vi "EMI_project_v5.vi"() -> ()   [LabVIEW 2020]
uses:
  <vilib>/Instr/_visa.llb/VISA Flush IO Buffer Mask.ctl
  <vilib>/Analysis/baseanly.llb/Mean (DBL).vi
  <vilib>/Instr/_visa.llb/VISA Configure Serial Port (Instr).vi
  <vilib>/Analysis/NI_AALBase.lvlib
panel:
  out "Numeric 2":dbl
  out "Numeric":dbl
  out "Boolean":bool
  out "Auto Mix LED":bool
  in  "stop 4":bool
  in  "stop 3":bool
  out "V_avg_live_CH02":dbl
  out "V_avg_live_CH01":dbl
  in  "Auto Mix ON/OFF":bool
  out "Take Average CH02":bool
  out "Take Average CH01":bool
  in  "Take Average CH 01":bool
  out "Voltage Peak CH02":dynamicdata(graph)
  out "Voltage Peak CH01":dynamicdata(graph)
  in  "stop 2":bool
  out "Voltage Thresould\n CH 2":dbl
  in  "Noise Thresould \nCH02":dbl
  in  "Take Average CH 2":bool
  out "Voltage Thresould\n CH 01":dbl
  in  "Noise Thresould\n CH01":dbl
  out "Fader 02 level":dbl
  out "Fader 01 level":dbl
  out "Gain Knob 02 level":dbl
  out "Gain knob 01 level":dbl
  out "manual mode led":bool
  out "Sound Balance Mode":bool
  in  "Gain Knob 02":dbl(knob) scale=0.0..300.0
  in  "Gain Knob 01":dbl(knob) scale=0.0..300.0
  in  "Fader 02 Slider":dbl(slide) scale=0.0..10.0
  in  "Fader 01 Slider":dbl(slide) scale=0.0..10.0
  out "Fader 02 Max":dbl
  out "Fader 01 Max":dbl
  in  "Calibrate":bool
  in  "stop":bool
  in  "VISA Resource":refnum<visa-resource-name>
  in  "?":bool
  in  "Gain 02":bool
  in  "?":bool
  in  "Gain 01":bool
  in  "?":bool
  in  "Fader 02":bool
  in  "?":bool
  in  "Fader 01":bool
  # "Automation System For Analog Audio Mixers"
  # "Calibration \nMode"
  # "Manual Mode"
  # "Sound Balance Mode"
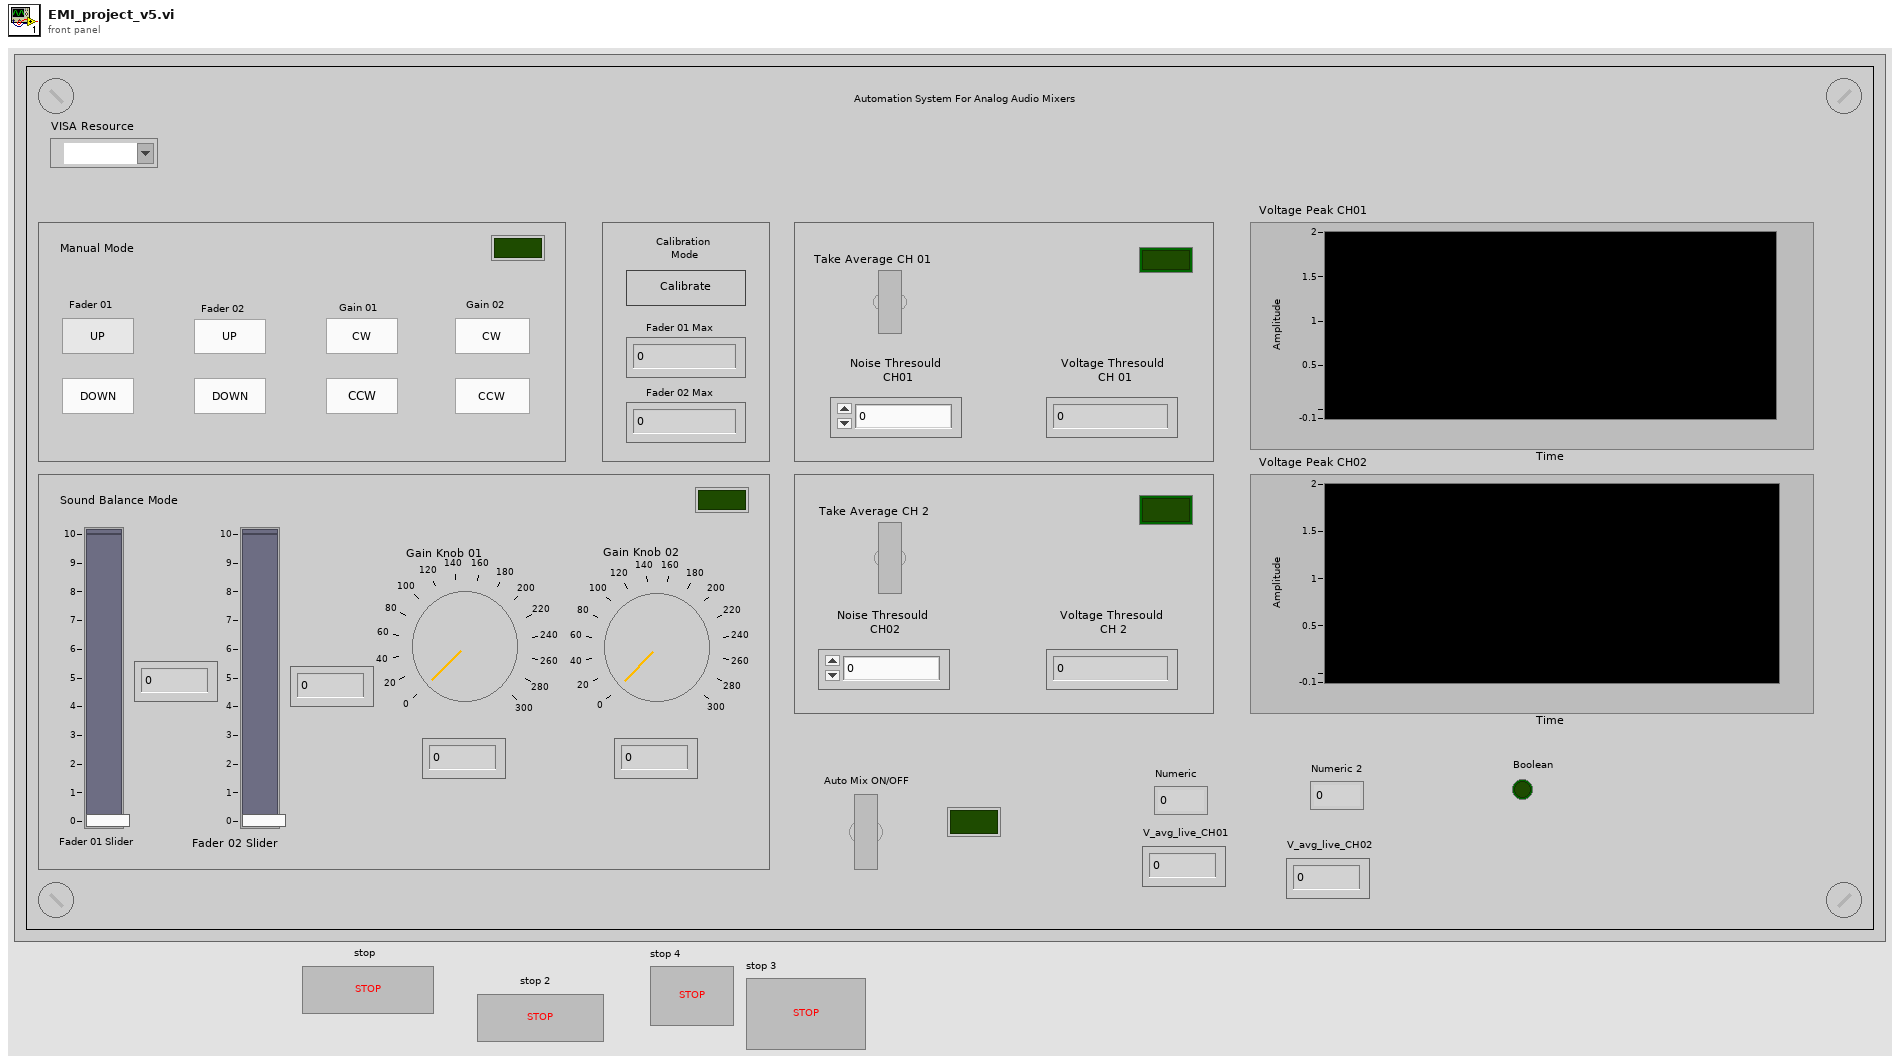
[diagram p1: front panel]
types:
  T1 = cluster{"Fader_Target_mm_1":dbl, "Fader_Target_mm_2":dbl, "Gain_Target_deg_1":dbl, "Gain_Target_deg_2":dbl}
  T2 = typedef "VISA Flush IO Buffer Mask.ctl" = u16
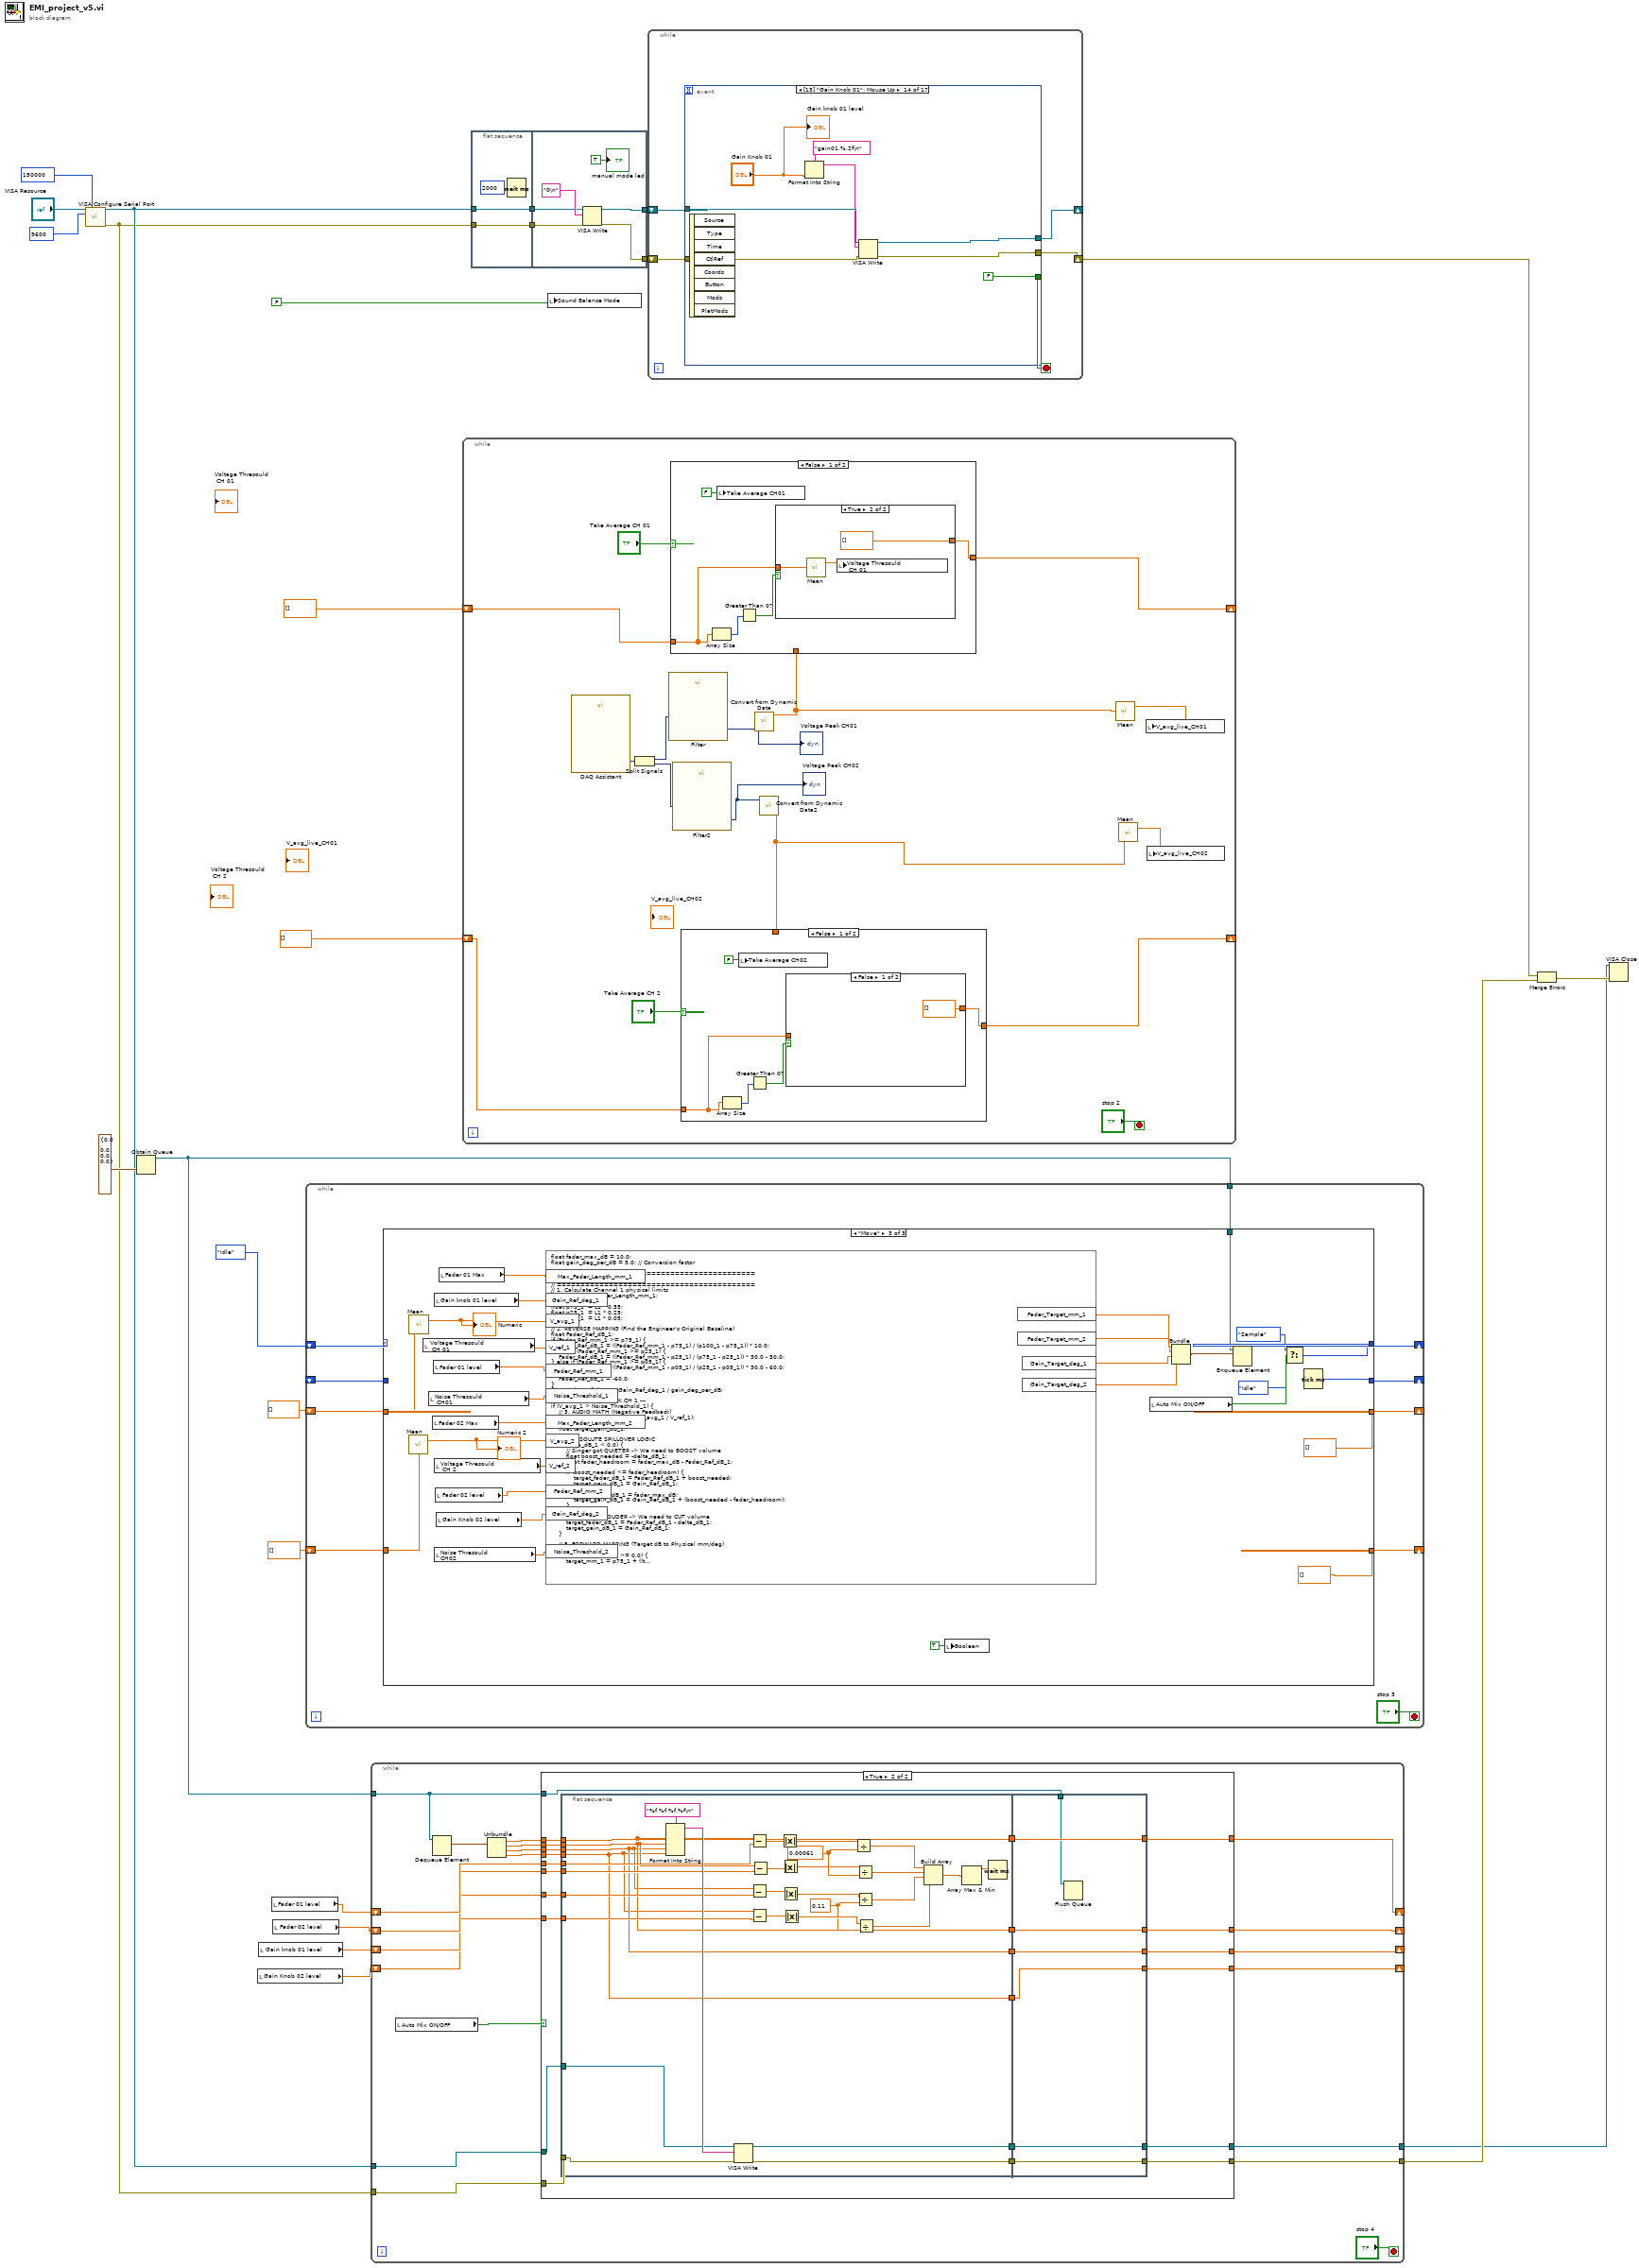
[diagram p0: block diagram]
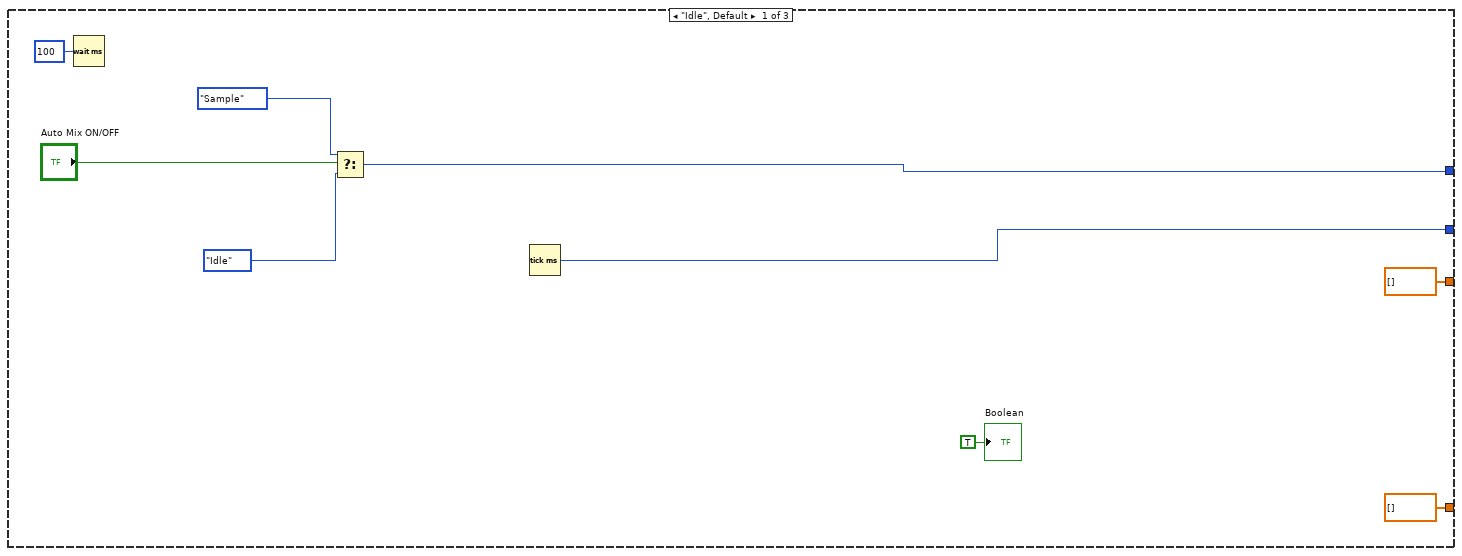
[diagram p3: hidden frame]
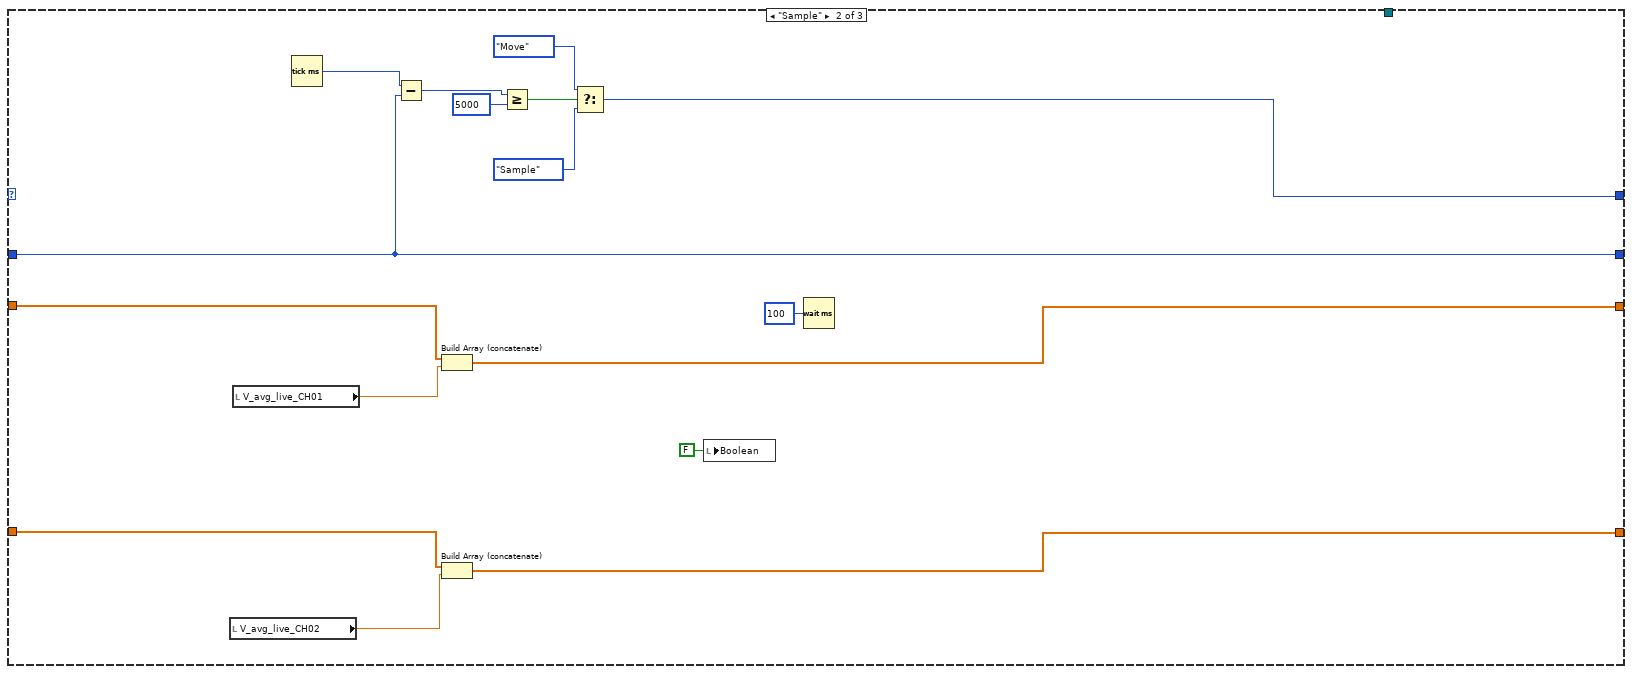
[diagram p4: hidden frame]
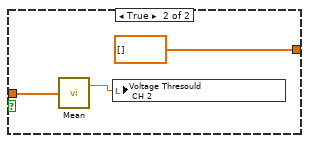
[diagram p5: hidden frame]
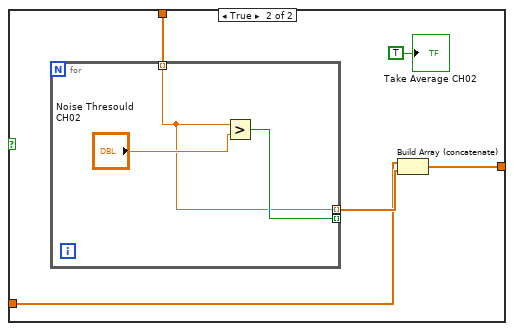
[diagram p6: hidden frame]
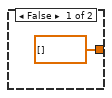
[diagram p7: hidden frame]
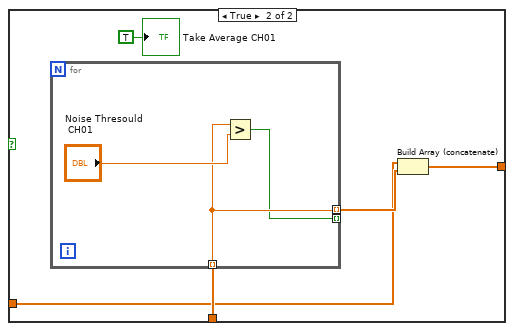
[diagram p8: hidden frame]
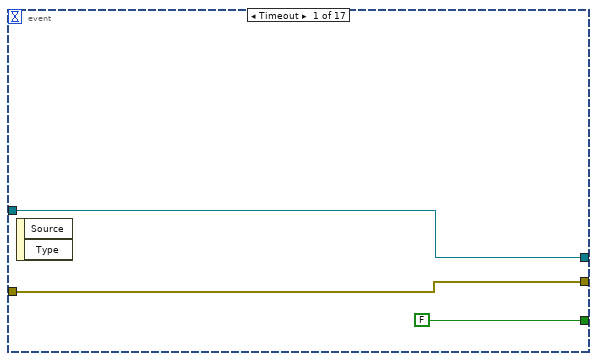
[diagram p9: hidden frame]
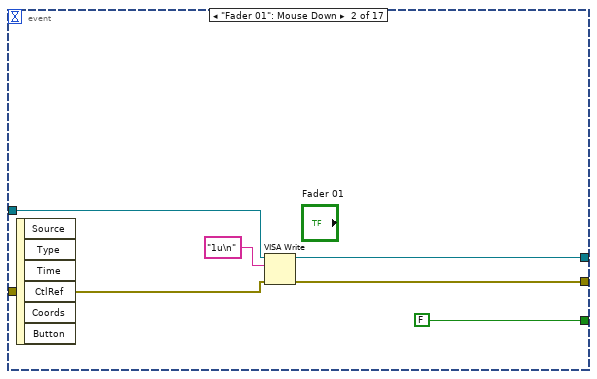
[diagram p10: hidden frame]
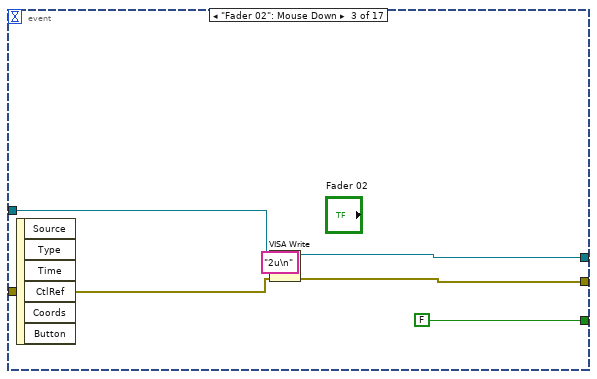
[diagram p11: hidden frame]
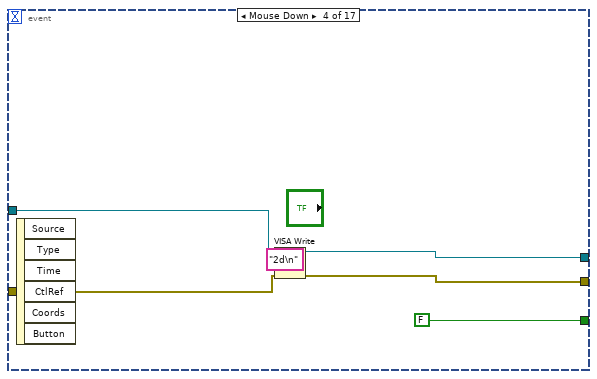
[diagram p12: hidden frame]
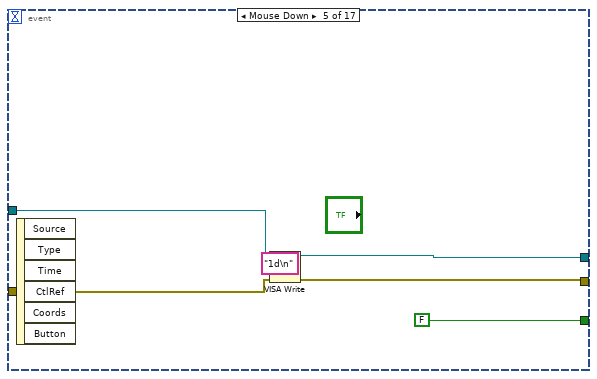
[diagram p13: hidden frame]
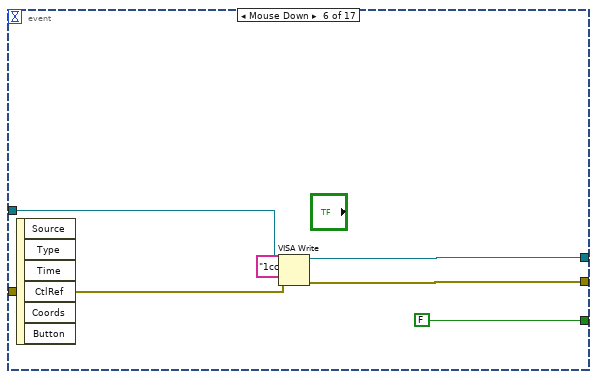
[diagram p14: hidden frame]
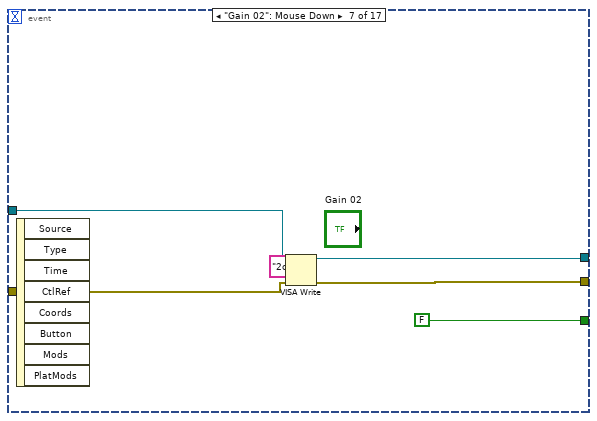
[diagram p15: hidden frame]
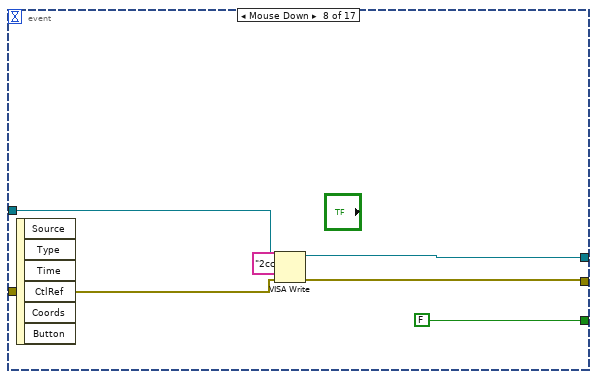
[diagram p16: hidden frame]
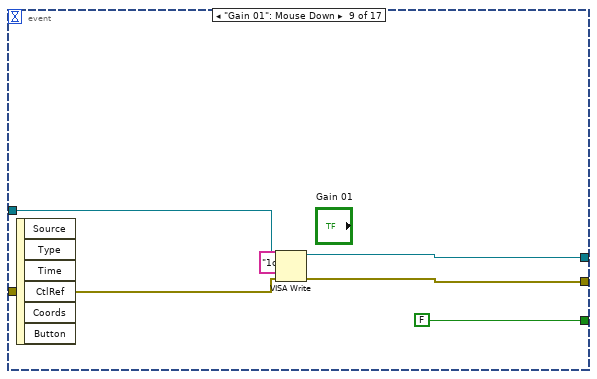
[diagram p17: hidden frame]
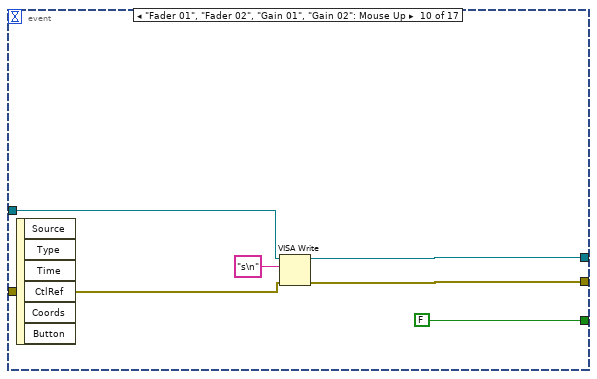
[diagram p18: hidden frame]
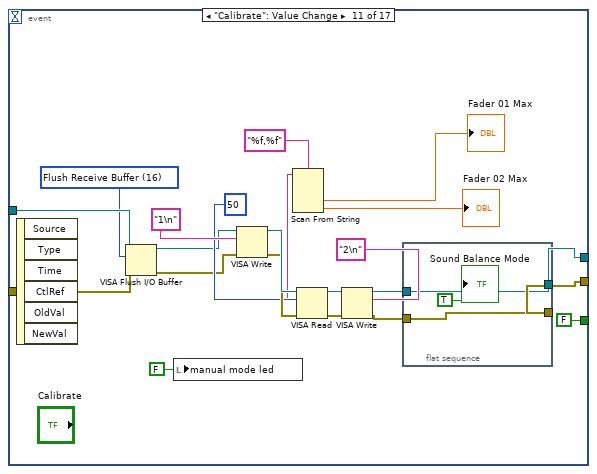
[diagram p19: hidden frame]
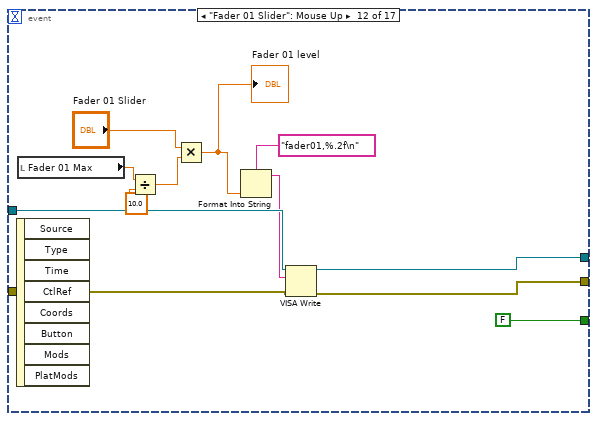
[diagram p20: hidden frame]
diagram:
  n1 = call-poly "VISA Configure Serial Port"("VISA resource name"="VISA Resource", "timeout (10sec)"=u32 150000, "baud rate (9600)"=u32 9600) -> ("VISA resource name out"=w11:refnum<visa-resource-name>, "error out"=w10:errorcluster)  [unwired: 11 in]
  n2 = Obtain Queue(element data type=T1 {"Fader_Target_mm_1"=0.0, "Fader_Target_mm_2"=0.0, "Gain_Target_deg_1"=0.0, "Gain_Target_deg_2"=0.0} ("output cluster")) -> (queue out=w12:refnum<queue>)  [unwired: 4 in, 2 out]
  n3 = local read "Gain Knob 02 level"() -> (w6:dbl)
  n4 = local read "Gain knob 01 level"() -> (w7:dbl)
  n5 = local read "Fader 01 level"() -> (w9:dbl)
  n6 = local read "Fader 02 level"() -> (w8:dbl)
  n7 = while {
    shift-right: [w34] -> _
    shift-left: enum16{"Idle", "Sample", "Move"}."Idle" -> [w35]
    shift-right: [w33] -> _
    shift-left: _ -> [w32]
    shift-right: [w30] -> _
    shift-left: dbl[] [] -> [w31]
    shift-right: [w29] -> _
    shift-left: dbl[] [] -> [w28]
    tunnel: w12 -> [w26]
    stop <- "stop 3" stop-if-true
    n8 = case shown="\"Move\"" w35 {
      tunnel: [w41 w54 w68] -> w34
      tunnel: [w36 w58 w63] -> w33
      tunnel: w32 -> [_ w58 _]
      tunnel: w31 -> [_ w53 w88]
      tunnel: [dbl[] [] w51 dbl[] []] -> w30
      tunnel: [dbl[] [] w48 dbl[] []] -> w29
      tunnel: w28 -> [_ w47 w85]
      tunnel: w26 -> [_ _ w73]
      frame "Idle", Default {
        n9 = Wait (ms)(milliseconds to wait=u32 100) -> ()  [unwired: 1 out]
        n10 = Select(t=enum16{"Idle", "Sample", "Move", "Wait"}."Sample", s="Auto Mix ON/OFF", f=enum16{"Idle", "Sample", "Move", "Wait"}."Idle") -> (s? t:f=w41:enum16{"Idle", "Sample", "Move", "Wait"})
        n11 = Tick Count (ms)() -> (millisecond timer value=w36:u32)
        "Boolean" <- TRUE ("Boolean")
      }
      frame "Sample" {
        n12 = local read "V_avg_live_CH02"() -> (w49:dbl)
        n13 = local read "V_avg_live_CH01"() -> (w52:dbl)
        n14 = Tick Count (ms)() -> (millisecond timer value=w45:u32)
        n15 = Subtract(x=w45, y=w58) -> (x-y=w60:u32)
        n16 = Build Array (concatenate)(w53, w52) -> (w51:dbl[])
        n17 = Build Array (concatenate)(w47, w49) -> (w48:dbl[])
        n18 = Greater Or Equal?(x=w60, y=u32 5000) -> (x >= y?=w57:bool)
        n19 = Select(t=enum16{"Idle", "Sample", "Move", "Wait"}."Move", s=w57, f=enum16{"Idle", "Sample", "Move", "Wait"}."Sample") -> (s? t:f=w54:enum16{"Idle", "Sample", "Move", "Wait"})
        n20 = local write "Boolean"(FALSE ("Boolean")) -> ()
        n21 = Wait (ms)(milliseconds to wait=u32 100) -> ()  [unwired: 1 out]
      }
      frame "Move" {
        n22 = call-poly <vilib>:"Mean.vi"("X"=w85) -> ("mean"=w61:dbl)  [unwired: 1 out]
        "Numeric 2" <- w61
        n23 = call-poly <vilib>:"Mean.vi"("X"=w88) -> ("mean"=w62:dbl)  [unwired: 1 out]
        "Numeric" <- w62
        n24 = local read "Voltage Thresould\n CH 01"() -> (w83:dbl)
        n25 = local read "Noise Thresould\n CH01"() -> (w66:dbl)
        n26 = local read "Fader 02 Max"() -> (w67:dbl)
        n27 = local read "Fader 01 level"() -> (w81:dbl)
        n28 = local read "Gain knob 01 level"() -> (w80:dbl)
        n29 = local read "Voltage Thresould\n CH 2"() -> (w82:dbl)
        n30 = local read "Noise Thresould \nCH02"() -> (w65:dbl)
        n31 = local read "Fader 02 level"() -> (w79:dbl)
        n32 = local read "Gain Knob 02 level"() -> (w78:dbl)
        n33 = local read "Fader 01 Max"() -> (w84:dbl)
        n34 = formula code="float fader_max_dB = 10.0;\nfloat gain_deg_per_dB = 5.0; // Conversion factor\n\n// ==========================================\n// CHANNEL 1 PROCESSING\n// ==========================================\n// 1. Calculate Channel 1 physical limits\nfloat L1 = Max_Fader_Length_mm_1; \nfloat p100_1 = L1;           \nfloat p75_1  = L1 * 0.55;    \nfloat p25_1  = L1 * 0.25;    \nfloat p05_1  = L1 * 0.05;    \n\n// 2. REVERSE MAPPING (Find the Engineer's Original Baseline)\nfloat Fader_Ref_dB_1;\nif (Fader_Ref_mm_1 >= p75_1) {\n    Fader_Ref_dB_1 = ((Fader_Ref_mm_1 - p75_1) / (p100_1 - p75_1)) * 10.0;\n} else if (Fader_Ref_mm_1 >= p25_1) {\n    Fader_Ref_dB_1 = ((Fader_Ref_mm_1 - p25_1) / (p75_1 - p25_1)) * 30.0 - 30.0;\n} else if (Fader_Ref_mm_1 >= p05_1) {\n    Fader_Ref_dB_1 = ((Fader_Ref_mm_1 - p05_1) / (p25_1 - p05_1)) * 30.0 - 60.0;\n} else {\n    Fader_Ref_dB_1 = -60.0; \n}\nfloat Gain_Ref_dB_1 = Gain_Ref_deg_1 / gain_deg_per_dB;\n\n// --- NOISE GATE CHECK CH 1 ---\nif (V_avg_1 > Noise_Threshold_1) {\n    // 3. AUDIO MATH (Negative Feedback)\n    float delta_dB_1 = 20 * log(V_avg_1 / V_ref_1);\n    float target_fader_dB_1;\n    float target_gain_dB_1;\n\n    // 4. ABSOLUTE SPILLOVER LOGIC\n    if (delta_dB_1 < 0.0) {\n        // Singer got QUIETER -> We need to BOOST volume\n        float boost_needed = -delta_dB_1; \n        float fader_headroom = fader_max_dB - Fader_Ref_dB_1;\n        \n        if (boost_needed <= fader_headroom) {\n            target_fader_dB_1 = Fader_Ref_dB_1 + boost_needed;\n            target_gain_dB_1 = Gain_Ref_dB_1;\n        } else {\n            target_fader_dB_1 = fader_max_dB;\n            target_gain_dB_1 = Gain_Ref_dB_1 + (boost_needed - fader_headroom);\n        }\n    } else {\n        // Singer got LOUDER -> We need to CUT volume\n        target_fader_dB_1 = Fader_Ref_dB_1 - delta_dB_1;\n        target_gain_dB_1 = Gain_Ref_dB_1;\n    }\n\n    // 5. FORWARD MAPPING (Target dB to Physical mm/deg)\n    float target_mm_1;\n    if (target_fader_dB_1 >= 0.0) {\n        target_mm_1 = p75_1 + ((target_fader_dB_1 - 0.0) / 10.0) * (p100_1 - p75_1);\n    } else if (target_fader_dB_1 >= -30.0) {\n        target_mm_1 = p25_1 + ((target_fader_dB_1 - (-30.0)) / 30.0) * (p75_1 - p25_1);\n    } else if (target_fader_dB_1 >= -60.0) {\n        target_mm_1 = p05_1 + ((target_fader_dB_1 - (-60.0)) / 30.0) * (p25_1 - p05_1);\n    } else {\n        target_mm_1 = 0.0; \n    }\n\n    Fader_Target_mm_1 = target_mm_1;\n    Gain_Target_deg_1 = target_gain_dB_1 * gain_deg_per_dB; \n\n    // 6. HARDWARE SAFETY CLAMP\n    if (Gain_Target_deg_1 > 300) { Gain_Target_deg_1 = 300; }\n    if (Gain_Target_deg_1 < 0.0) { Gain_Target_deg_1 = 0.0; }\n\n} else {\n    // AUDIO IS BELOW NOISE THRESHOLD\n    // Do nothing: lock the targets to the current physical positions\n    Fader_Target_mm_1 = Fader_Ref_mm_1;\n    Gain_Target_deg_1 = Gain_Ref_deg_1;\n}\n\n\n// ==========================================\n// CHANNEL 2 PROCESSING\n// ==========================================\n// 1. Calculate Channel 2 physical limits\nfloat L2 = Max_Fader_Length_mm_2; \nfloat p100_2 = L2;           \nfloat p75_2  = L2 * 0.55;    \nfloat p25_2  = L2 * 0.25;    \nfloat p05_2  = L2 * 0.05;    \n\n// 2. REVERSE MAPPING (Find the Engineer's Original Baseline)\nfloat Fader_Ref_dB_2;\nif (Fader_Ref_mm_2 >= p75_2) {\n    Fader_Ref_dB_2 = ((Fader_Ref_mm_2 - p75_2) / (p100_2 - p75_2)) * 10.0;\n} else if (Fader_Ref_mm_2 >= p25_2) {\n    Fader_Ref_dB_2 = ((Fader_Ref_mm_2 - p25_2) / (p75_2 - p25_2)) * 30.0 - 30.0;\n} else if (Fader_Ref_mm_2 >= p05_2) {\n    Fader_Ref_dB_2 = ((Fader_Ref_mm_2 - p05_2) / (p25_2 - p05_2)) * 30.0 - 60.0;\n} else {\n    Fader_Ref_dB_2 = -60.0; \n}\nfloat Gain_Ref_dB_2 = Gain_Ref_deg_2 / gain_deg_per_dB;\n\n// --- NOISE GATE CHECK CH 2 ---\nif (V_avg_2 > Noise_Threshold_2) {\n    // 3. AUDIO MATH (Negative Feedback)\n    float delta_dB_2 = 20 * log(V_avg_2 / V_ref_2);\n    float target_fader_dB_2;\n    float target_gain_dB_2;\n\n    // 4. ABSOLUTE SPILLOVER LOGIC\n    if (delta_dB_2 < 0.0) {\n        // Singer got QUIETER -> We need to BOOST volume\n        float boost_needed = -delta_dB_2; \n        float fader_headroom = fader_max_dB - Fader_Ref_dB_2;\n        \n        if (boost_needed <= fader_headroom) {\n            target_fader_dB_2 = Fader_Ref_dB_2 + boost_needed;\n            target_gain_dB_2 = Gain_Ref_dB_2;\n        } else {\n            target_fader_dB_2 = fader_max_dB;\n            target_gain_dB_2 = Gain_Ref_dB_2 + (boost_needed - fader_headroom);\n        }\n    } else {\n        // Singer got LOUDER -> We need to CUT volume\n        target_fader_dB_2 = Fader_Ref_dB_2 - delta_dB_2;\n        target_gain_dB_2 = Gain_Ref_dB_2;\n    }\n\n    // 5. FORWARD MAPPING (Target dB to Physical mm/deg)\n    float target_mm_2;\n    if (target_fader_dB_2 >= 0.0) {\n        target_mm_2 = p75_2 + ((target_fader_dB_2 - 0.0) / 10.0) * (p100_2 - p75_2);\n    } else if (target_fader_dB_2 >= -30.0) {\n        target_mm_2 = p25_2 + ((target_fader_dB_2 - (-30.0)) / 30.0) * (p75_2 - p25_2);\n    } else if (target_fader_dB_2 >= -60.0) {\n        target_mm_2 = p05_2 + ((target_fader_dB_2 - (-60.0)) / 30.0) * (p25_2 - p05_2);\n    } else {\n        target_mm_2 = 0.0; \n    }\n\n    Fader_Target_mm_2 = target_mm_2;\n    Gain_Target_deg_2 = target_gain_dB_2 * gain_deg_per_dB; \n\n    // 6. HARDWARE SAFETY CLAMP\n    if (Gain_Target_deg_2 > 300) { Gain_Target_deg_2 = 300; }\n    if (Gain_Target_deg_2 < 0.0) { Gain_Target_deg_2 = 0.0; }\n\n} else {\n    // AUDIO IS BELOW NOISE THRESHOLD\n    // Do nothing: lock the targets to the current physical positions\n    Fader_Target_mm_2 = Fader_Ref_mm_2;\n    Gain_Target_deg_2 = Gain_Ref_deg_2;\n}"("Max_Fader_Length_mm_1"=w84, "Max_Fader_Length_mm_2"=w67, "V_avg_1"=w62, "V_ref_1"=w83, "V_avg_2"=w61, "V_ref_2"=w82, "Fader_Ref_mm_1"=w81, "Fader_Ref_mm_2"=w79, "Gain_Ref_deg_1"=w80, "Gain_Ref_deg_2"=w78, "Noise_Threshold_1"=w66, "Noise_Threshold_2"=w65) -> ("Fader_Target_mm_1"=w77:dbl, "Fader_Target_mm_2"=w76:dbl, "Gain_Target_deg_1"=w75:dbl, "Gain_Target_deg_2"=w74:dbl)
        n35 = local write "Boolean"(TRUE ("Boolean")) -> ()
        n36 = local read "Auto Mix ON/OFF"() -> (w71:bool)
        n37 = Bundle("Fader_Target_mm_1"=w77, "Fader_Target_mm_2"=w76, "Gain_Target_deg_1"=w75, "Gain_Target_deg_2"=w74) -> (w72:T1)  [unwired: 1 in]
        n38 = Enqueue Element(queue=w73, element=w72) -> ()  [unwired: 2 in, 3 out]
        n39 = Select(t=enum16{"Idle", "Sample", "Move", "Wait"}."Sample", s=w71, f=enum16{"Idle", "Sample", "Move", "Wait"}."Idle") -> (s? t:f=w68:enum16{"Idle", "Sample", "Move", "Wait"})
        n40 = Tick Count (ms)() -> (millisecond timer value=w63:u32)
      }
    }
  }
  n41 = while {
    tunnel: w12 -> [w89]
    tunnel: w11 -> [w102]
    tunnel: w10 -> [w101]
    shift-right: [w96] -> _
    shift-left: w9 -> [w100]
    shift-right: [w95] -> _
    shift-left: w8 -> [w99]
    shift-right: [w94] -> _
    shift-left: w7 -> [w98]
    shift-right: [w93] -> _
    shift-left: w6 -> [w97]
    tunnel: [w92] -> w2
    tunnel: [w91] -> w5
    stop <- "stop 4" stop-if-true
    n42 = local read "Auto Mix ON/OFF"() -> (w107:bool)
    n43 = Dequeue Element(queue=w89) -> (element=w108:T1)  [unwired: 2 in, 3 out]
    n44 = Unbundle(w108) -> ("Fader_Target_mm_1"=w106:dbl, "Fader_Target_mm_2"=w105:dbl, "Gain_Target_deg_1"=w104:dbl, "Gain_Target_deg_2"=w103:dbl)
    n45 = case shown="True" w107 {
      tunnel: w106 -> [_ w137]
      tunnel: w105 -> [_ w136]
      tunnel: w104 -> [_ w135]
      tunnel: w103 -> [_ w134]
      tunnel: w102 -> [w110 w132]
      tunnel: w101 -> [w109 w133]
      tunnel: w100 -> [w114 w131]
      tunnel: w99 -> [w113 w130]
      tunnel: w98 -> [w112 w129]
      tunnel: w97 -> [w111 w128]
      tunnel: [w114 w126] -> w96
      tunnel: [w113 w125] -> w95
      tunnel: [w112 w123] -> w94
      tunnel: [w111 w120] -> w93
      tunnel: [w110 w119] -> w92
      tunnel: [w109 w117] -> w91
      tunnel: w89 -> [_ w115]
      frame False {
      }
      frame True {
        n46 = flat-sequence {
          tunnel: w137 -> [w145]
          tunnel: w136 -> [w144]
          tunnel: w135 -> [w143]
          tunnel: w134 -> [w142]
          tunnel: w133 -> [w138]
          tunnel: w132 -> [w139]
          tunnel: w131 -> [w165]
          tunnel: w130 -> [w164]
          tunnel: w129 -> [w163]
          tunnel: w128 -> [w162]
          tunnel: [w145] -> w127
          tunnel: [w144] -> w124
          tunnel: [w143] -> w122
          tunnel: [w142] -> w121
          tunnel: [w141] -> w118
          tunnel: [w140] -> w116
          tunnel: w127 -> [w174]
          tunnel: [w174] -> w126
          tunnel: [w173] -> w125
          tunnel: w124 -> [w173]
          tunnel: [w172] -> w123
          tunnel: w122 -> [w172]
          tunnel: w121 -> [w171]
          tunnel: [w171] -> w120
          tunnel: [w170] -> w119
          tunnel: w118 -> [w170]
          tunnel: [w169] -> w117
          tunnel: w116 -> [w169]
          tunnel: w115 -> [w168]
          frame #0 {
            w148 = 0.11 ("y")
            w157 = 0.00061 ("y")
            n47 = Format Into String(format string="%f,%f,%f,%f\n", w145, w144, w143, w142) -> (resulting string=w166:string)  [unwired: 2 in, 1 out]
            n48 = VISA Write(VISA resource name=w139, write buffer=w166, error in (no error)=w138) -> (VISA resource name out=w141:refnum<visa-resource-name>, error out=w140:errorcluster)  [unwired: 1 out]
            n49 = Subtract(x=w145, y=w165) -> (x-y=w161:dbl)
            n50 = Subtract(x=w143, y=w163) -> (x-y=w159:dbl)
            n51 = Subtract(x=w142, y=w162) -> (x-y=w158:dbl)
            n52 = Subtract(x=w144, y=w164) -> (x-y=w160:dbl)
            n53 = Absolute Value(x=w161) -> (abs(x)=w156:dbl)
            n54 = Absolute Value(x=w160) -> (abs(x)=w155:dbl)
            n55 = Absolute Value(x=w159) -> (abs(x)=w154:dbl)
            n56 = Absolute Value(x=w158) -> (abs(x)=w153:dbl)
            n57 = Divide(x=w156, y=w157) -> (x/y=w152:dbl)
            n58 = Divide(x=w155, y=w157) -> (x/y=w151:dbl)
            n59 = Divide(x=w154, y=w148) -> (x/y=w150:dbl)
            n60 = Divide(x=w153, y=w148) -> (x/y=w149:dbl)
            n61 = Build Array(w152, w151, w150, w149) -> (w147:dbl[])
            n62 = Array Max & Min(array=w147) -> (max value=w146:dbl)  [unwired: 3 out]
            n63 = Wait (ms)(milliseconds to wait=w146) -> ()  [unwired: 1 out]
          }
          frame #1 {
            n64 = Flush Queue(queue=w168) -> ()  [unwired: 1 in, 3 out]
          }
        }
      }
    }
  }
  n65 = while {
    shift-right: [w185] -> _
    shift-left: dbl[] [] -> [w186]
    shift-right: [w183] -> _
    shift-left: dbl[] [] -> [w182]
    stop <- "stop 2" stop-if-true
    n66 = call "DAQ Assistant"() -> ("data"=w189:dynamicdata)  [unwired: 16 in, 3 out]
    n67 = Split Signals(w189) -> (w188:dynamicdata, w187:dynamicdata)  [unwired: 2 in]
    n68 = call "Filter"("Signal"=w188) -> ("Filtered Signal"=w180:dynamicdata)  [unwired: 9 in, 1 out]
    "Voltage Peak CH01" <- w180
    n69 = call "Filter2"("Signal"=w187) -> ("Filtered Signal"=w179:dynamicdata)  [unwired: 9 in, 1 out]
    "Voltage Peak CH02" <- w179
    n70 = call "Convert from Dynamic Data"("Dynamic Data Type"=w180) -> ("Array"=w176:dbl[])  [unwired: 3 in]
    n71 = case shown="False" "Take Average CH 01" {
      tunnel: w176 -> [_ w221]
      tunnel: w186 -> [w210 w218]
      tunnel: [w209 w219] -> w185
      frame False {
        n72 = Array Size(array=w210) -> (size(s)=w212:i32)
        n73 = local write "Take Average CH01"(FALSE ("Take Average CH01")) -> ()
        n74 = Greater Than 0?(x=w212) -> (x > 0?=w211:bool)
        n75 = case shown="True" w211 {
          tunnel: w210 -> [_ w216]
          tunnel: [dbl[] [] dbl[] []] -> w209
          frame False {
          }
          frame True {
            n76 = call-poly <vilib>:"Mean.vi"("X"=w216) -> ("mean"=w215:dbl)  [unwired: 1 out]
            n77 = local write "Voltage Thresould\n CH 01"(w215) -> ()
          }
        }
      }
      frame True {
        n78 = for {
          tunnel: w221 -> [w223] mode=indexing
          tunnel: [w223] -> w220 mode=indexing if=w222
          tunnel: [w222] -> _ mode=indexing
          n79 = Greater?(x=w223, y="Noise Thresould\n CH01") -> (0:w222:bool)
        }
        n80 = Build Array (concatenate)(w218, w220) -> (w219:dbl[])
        "Take Average CH01" <- TRUE ("Take Average CH01")
      }
    }
    n81 = call "Convert from Dynamic Data2"("Dynamic Data Type"=w179) -> ("Array"=w175:dbl[])  [unwired: 3 in]
    n82 = case shown="False" "Take Average CH 2" {
      tunnel: w182 -> [w193 w203]
      tunnel: [w192 w202] -> w183
      tunnel: w175 -> [_ w201]
      frame False {
        n83 = Array Size(array=w193) -> (size(s)=w195:i32)
        n84 = local write "Take Average CH02"(FALSE ("Take Average CH02")) -> ()
        n85 = Greater Than 0?(x=w195) -> (x > 0?=w194:bool)
        n86 = case shown="False" w194 {
          tunnel: w193 -> [_ w199]
          tunnel: [dbl[] [] dbl[] []] -> w192
          frame False {
          }
          frame True {
            n87 = call-poly <vilib>:"Mean.vi"("X"=w199) -> ("mean"=w198:dbl)  [unwired: 1 out]
            n88 = local write "Voltage Thresould\n CH 2"(w198) -> ()
          }
        }
      }
      frame True {
        n89 = for {
          tunnel: [w205] -> w204 mode=indexing if=w206
          tunnel: [w206] -> _ mode=indexing
          tunnel: w201 -> [w205] mode=indexing
          n90 = Greater?(x=w205, y="Noise Thresould \nCH02") -> (0:w206:bool)
        }
        n91 = Build Array (concatenate)(w203, w204) -> (w202:dbl[])
        "Take Average CH02" <- TRUE ("Take Average CH02")
      }
    }
    n92 = call-poly <vilib>:"Mean.vi"("X"=w176) -> ("mean"=w178:dbl)  [unwired: 1 out]
    n93 = call-poly <vilib>:"Mean.vi"("X"=w175) -> ("mean"=w177:dbl)  [unwired: 1 out]
    n94 = local write "V_avg_live_CH01"(w178) -> ()
    n95 = local write "V_avg_live_CH02"(w177) -> ()
  }
  n96 = flat-sequence {
    tunnel: w10 -> [w226]
    tunnel: w11 -> [w227]
    tunnel: [w227] -> w21
    tunnel: [w226] -> w20
    tunnel: [w232] -> w23
    tunnel: [w231] -> w22
    tunnel: w21 -> [w230]
    tunnel: w20 -> [w229]
    frame #0 {
      n97 = Wait (ms)(milliseconds to wait=u32 2000) -> ()  [unwired: 1 out]
    }
    frame #1 {
      n98 = VISA Write(VISA resource name=w230, write buffer="0\n", error in (no error)=w229) -> (VISA resource name out=w232:refnum<visa-resource-name>, error out=w231:errorcluster)  [unwired: 1 out]
      "manual mode led" <- TRUE
    }
  }
  n99 = local write "Sound Balance Mode"(FALSE) -> ()
  n100 = while {
    shift-right: [w236] -> _
    shift-left: w23 -> [w238]
    shift-right: [w235] -> w4
    shift-left: w22 -> [w237]
    stop <- w234 stop-if-true
    n101 = event shown="[13] \"Gain Knob 01\": Mouse Up" {
      selector: _ -> [_ _ _ _ _ _ _ _ _ _ _ _ _ _ _ _ _]
      dyn-events: _ -> [_ _ _ _ _ _ _ _ _ _ _ _ _ _ _ _ _]
      timeout: _ -> [_ _ _ _ _ _ _ _ _ _ _ _ _ _ _ _ _]
      tunnel: w238 -> [w241 w247 w251 w257 w265 w268 w275 w281 w287 w293 w309 w327 w338 w351 w358 w364 w382]
      tunnel: w237 -> [w240 w246 w250 w256 w264 w269 w274 w280 w286 w292 w308 w326 w337 w350 w357 w362 w381]
      tunnel: [w241 w244 w253 w259 w262 w271 w277 w283 w289 w295 w300 w323 w335 w348 w355 w363 w382] -> w236
      tunnel: [w240 w243 w252 w258 w263 w270 w276 w282 w288 w294 w297 w325 w336 w349 w356 w361 w381] -> w235
      tunnel: [FALSE FALSE FALSE FALSE FALSE FALSE FALSE FALSE FALSE FALSE FALSE FALSE FALSE FALSE FALSE FALSE TRUE] -> w234
      event Timeout {
        n102 = event-data() -> ()  [unwired: 1 in, 2 out]
      }
      event "Fader 01": Mouse Down {
        n103 = event-data() -> ()  [unwired: 1 in, 6 out]
        n104 = VISA Write(VISA resource name=w247, write buffer="1u\n", error in (no error)=w246) -> (VISA resource name out=w244:refnum<visa-resource-name>, error out=w243:errorcluster)  [unwired: 1 out]
      }
      event "Fader 02": Mouse Down {
        n105 = event-data() -> ()  [unwired: 1 in, 6 out]
        n106 = VISA Write(VISA resource name=w251, write buffer="2u\n", error in (no error)=w250) -> (VISA resource name out=w253:refnum<visa-resource-name>, error out=w252:errorcluster)  [unwired: 1 out]
      }
      event Mouse Down {
        n107 = event-data() -> ()  [unwired: 1 in, 6 out]
        n108 = VISA Write(VISA resource name=w257, write buffer="2d\n", error in (no error)=w256) -> (VISA resource name out=w259:refnum<visa-resource-name>, error out=w258:errorcluster)  [unwired: 1 out]
      }
      event Mouse Down {
        n109 = event-data() -> ()  [unwired: 1 in, 6 out]
        n110 = VISA Write(VISA resource name=w265, write buffer="1d\n", error in (no error)=w264) -> (VISA resource name out=w262:refnum<visa-resource-name>, error out=w263:errorcluster)  [unwired: 1 out]
      }
      event Mouse Down {
        n111 = event-data() -> ()  [unwired: 1 in, 6 out]
        n112 = VISA Write(VISA resource name=w268, write buffer="1ccw\n", error in (no error)=w269) -> (VISA resource name out=w271:refnum<visa-resource-name>, error out=w270:errorcluster)  [unwired: 1 out]
      }
      event "Gain 02": Mouse Down {
        n113 = event-data() -> ()  [unwired: 1 in, 8 out]
        n114 = VISA Write(VISA resource name=w275, write buffer="2cw\n", error in (no error)=w274) -> (VISA resource name out=w277:refnum<visa-resource-name>, error out=w276:errorcluster)  [unwired: 1 out]
      }
      event Mouse Down {
        n115 = event-data() -> ()  [unwired: 1 in, 6 out]
        n116 = VISA Write(VISA resource name=w281, write buffer="2ccw\n", error in (no error)=w280) -> (VISA resource name out=w283:refnum<visa-resource-name>, error out=w282:errorcluster)  [unwired: 1 out]
      }
      event "Gain 01": Mouse Down {
        n117 = event-data() -> ()  [unwired: 1 in, 6 out]
        n118 = VISA Write(VISA resource name=w287, write buffer="1cw\n", error in (no error)=w286) -> (VISA resource name out=w289:refnum<visa-resource-name>, error out=w288:errorcluster)  [unwired: 1 out]
      }
      event "Fader 01", "Fader 02", "Gain 01", "Gain 02": Mouse Up {
        n119 = event-data() -> ()  [unwired: 1 in, 6 out]
        n120 = VISA Write(VISA resource name=w293, write buffer="s\n", error in (no error)=w292) -> (VISA resource name out=w295:refnum<visa-resource-name>, error out=w294:errorcluster)  [unwired: 1 out]
      }
      event "Calibrate": Value Change {
        w305 = T2 16 items=["Flush Receive Buffer"=16, "Write Transmit Buffer to Device"=32, "Flush Receive Buffer (No I/O)"=64, "Flush Transmit Buffer"=128] ("Mask")
        n121 = event-data() -> ()  [unwired: 1 in, 6 out]
        n122 = VISA Flush I/O Buffer(VISA resource name=w309, mask (16)=w305, error in (no error)=w308) -> (VISA resource name out=w307:refnum<visa-resource-name>, error out=w306:errorcluster)
        n123 = local write "manual mode led"(FALSE ("manual mode led")) -> ()
        n124 = VISA Write(VISA resource name=w307, write buffer="1\n", error in (no error)=w306) -> (VISA resource name out=w316:refnum<visa-resource-name>, error out=w315:errorcluster)  [unwired: 1 out]
        n125 = VISA Read(VISA resource name=w316, byte count=u32 50, error in (no error)=w315) -> (VISA resource name out=w304:refnum<visa-resource-name>, read buffer=w313:string, error out=w303:errorcluster)  [unwired: 1 out]
        n126 = Scan From String(format string="%f,%f", input string=w313) -> (output 1=→"Fader 01 Max":dbl, output 2=→"Fader 02 Max":dbl)  [unwired: 4 in, 3 out]
        n127 = VISA Write(VISA resource name=w304, write buffer="2\n", error in (no error)=w303) -> (VISA resource name out=w299:refnum<visa-resource-name>, error out=w298:errorcluster)  [unwired: 1 out]
        n128 = flat-sequence {
          tunnel: [w319] -> w300
          tunnel: w299 -> [w319]
          tunnel: w298 -> [w318]
          tunnel: [w318] -> w297
          frame #0 {
            "Sound Balance Mode" <- TRUE
          }
        }
      }
      event "Fader 01 Slider": Mouse Up {
        n129 = event-data() -> ()  [unwired: 1 in, 8 out]
        n130 = local read "Fader 01 Max"() -> (w331:dbl)
        n131 = Divide(x=w331, y=10.0) -> (x/y=w328:dbl)
        n132 = Multiply(x="Fader 01 Slider", y=w328) -> (x*y=w321:dbl)
        "Fader 01 level" <- w321
        n133 = Format Into String(format string="fader01,%.2f\n", w321) -> (resulting string=w322:string)  [unwired: 2 in, 1 out]
        n134 = VISA Write(VISA resource name=w327, write buffer=w322, error in (no error)=w326) -> (VISA resource name out=w323:refnum<visa-resource-name>, error out=w325:errorcluster)  [unwired: 1 out]
      }
      event "Fader 02 Slider": Mouse Up {
        n135 = event-data() -> ()  [unwired: 1 in, 8 out]
        n136 = local read "Fader 02 Max"() -> (w344:dbl)
        n137 = Divide(x=w344, y=10.0) -> (x/y=w341:dbl)
        n138 = Multiply(x="Fader 02 Slider", y=w341) -> (x*y=w333:dbl)
        "Fader 02 level" <- w333
        n139 = Format Into String(format string="fader02,%.2f\n", w333) -> (resulting string=w339:string)  [unwired: 2 in, 1 out]
        n140 = VISA Write(VISA resource name=w338, write buffer=w339, error in (no error)=w337) -> (VISA resource name out=w335:refnum<visa-resource-name>, error out=w336:errorcluster)  [unwired: 1 out]
      }
      event "Gain Knob 01": Mouse Up {
        n141 = event-data() -> ()  [unwired: 1 in, 8 out]
        n142 = Format Into String(format string="gain01,%.2f\n", "Gain Knob 01") -> (resulting string=w347:string)  [unwired: 2 in, 1 out]
        n143 = VISA Write(VISA resource name=w351, write buffer=w347, error in (no error)=w350) -> (VISA resource name out=w348:refnum<visa-resource-name>, error out=w349:errorcluster)  [unwired: 1 out]
        "Gain knob 01 level" <- "Gain Knob 01"
      }
      event "Gain Knob 02": Mouse Up {
        n144 = event-data() -> ()  [unwired: 1 in, 8 out]
        n145 = Format Into String(format string="gain02,%.2f\n", "Gain Knob 02") -> (resulting string=w359:string)  [unwired: 2 in, 1 out]
        n146 = VISA Write(VISA resource name=w358, write buffer=w359, error in (no error)=w357) -> (VISA resource name out=w355:refnum<visa-resource-name>, error out=w356:errorcluster)  [unwired: 1 out]
        "Gain Knob 02 level" <- "Gain Knob 02"
      }
      event "Auto Mix ON/OFF": Value Change {
        n147 = event-data() -> ()  [unwired: 1 in, 6 out]
        n148 = local read "Auto Mix ON/OFF"() -> (w366:bool)
        n149 = case shown="False" w366 {
          tunnel: w364 -> [w370 w380]
          tunnel: [w372 w379] -> w363
          tunnel: w362 -> [w373 w378]
          tunnel: [w371 w377] -> w361
          frame False {
            n150 = local write "Sound Balance Mode"(TRUE ("Sound Balance Mode")) -> ()
            n151 = VISA Write(VISA resource name=w370, write buffer="2\n", error in (no error)=w373) -> (VISA resource name out=w372:refnum<visa-resource-name>, error out=w371:errorcluster)  [unwired: 1 out]
            n152 = local write "Auto Mix LED"(FALSE ("Auto Mix LED")) -> ()
          }
          frame True {
            n153 = VISA Write(VISA resource name=w380, write buffer="3\n", error in (no error)=w378) -> (VISA resource name out=w379:refnum<visa-resource-name>, error out=w377:errorcluster)  [unwired: 1 out]
            n154 = local write "Sound Balance Mode"(FALSE ("Sound Balance Mode")) -> ()
            "Auto Mix LED" <- TRUE ("Auto Mix LED")
          }
        }
      }
      event "stop": Value Change {
        n155 = event-data() -> ()  [unwired: 1 in, 6 out]
      }
    }
  }
  n156 = Merge Errors(w4, w5) -> (w3:errorcluster)
  n157 = VISA Close(VISA resource name=w2, error in (no error)=w3) -> ()  [unwired: 1 out]
